vi "GetSampleTime.vi"(11 "所有记录输入":string[](array[string])) -> (2 "area_name":string, 3 "所有记录输出":string[][](array[string]))   [LabVIEW 2014, in "cyy.lvlib"]
uses:
  CYY/cyy.lvlib
  DataBase.lvlib
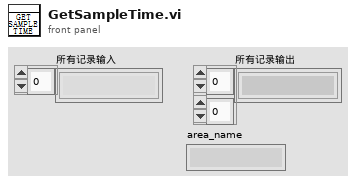
[diagram p1: front panel]
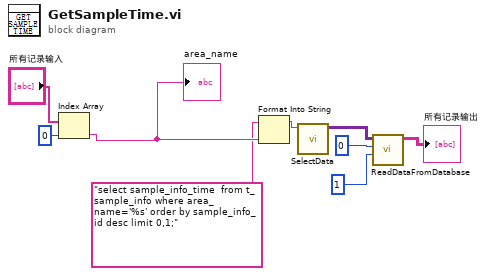
[diagram p0: block diagram]
diagram:
  n1 = Index Array(array="所有记录输入", index=0 ("索引")) -> (element=w4:string)
  "area_name" <- w4
  n2 = Format Into String(format string="select sample_info_time  from t_sample_info where area_name='%s' order by sample_info_id desc limit 0,1;", w4) -> (resulting string=w5:string)  [unwired: 2 in, 1 out]
  n3 = call "SelectData.vi"("SQL query"=w5) -> ("recordset data"=w6:variant[][])  [unwired: 7 in, 1 out]
  n4 = call "ReadDataFromDatabase.vi"("长度"=1, "index"=0, "recordset data"=w6) -> ("所有记录"=→"所有记录输出":string[][])  [unwired: 7 in, 1 out]
